vi "Coherent laser status decode.vi"(11 "I/p String":string) -> (2 "Boolean":bool, 3 "String":string)   [LabVIEW 2020]
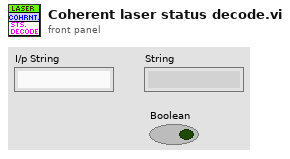
[diagram p1: front panel]
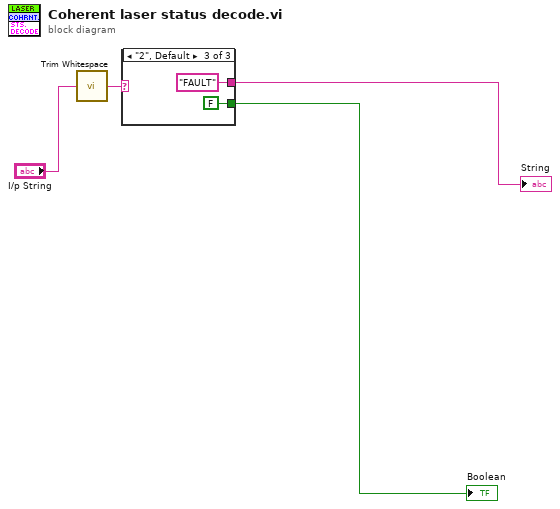
[diagram p0: block diagram]
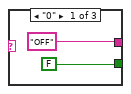
[diagram p2: hidden frame]
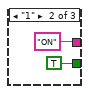
[diagram p3: hidden frame]
diagram:
  n1 = call <vilib>:"Trim Whitespace.vi"("string"="I/p String") -> ("trimmed string"=w2:string)  [unwired: 1 in]
  n2 = case shown="\"2\", Default" w2 {
    tunnel: ["OFF" "ON" "FAULT"] -> w3
    tunnel: [FALSE TRUE FALSE] -> w4
    frame "0" {
    }
    frame "1" {
    }
    frame "2", Default {
    }
  }
  "Boolean" <- w4
  "String" <- w3
